vi "FC_Get_Target_Info.vi"(7 "Target":T1, 8 "Error In":errorcluster, 9 "Desired Target":string, 10 "Array of Targets":string[](array[string]), 11 "Target XML":string) -> (0 "error out":errorcluster, 2 "Target Info":string)   [LabVIEW 2013, in "FC_FIRST Client.lvlib"]
doc: "This VI returns all of the information about a specified target"
uses:
  FC_FIRST Client.lvlib
  FC_Target.ctl
  <vilib>/regexp/Match Regular Expression.xnode
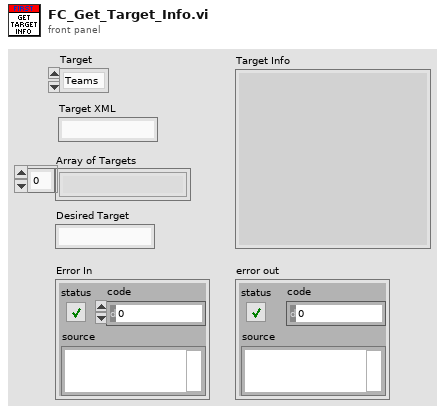
[diagram p1: front panel]
types:
  T1 = typedef "FC_FIRST Client.lvlib/FC_Target.ctl" = enum16{"Teams", "Competitions"}
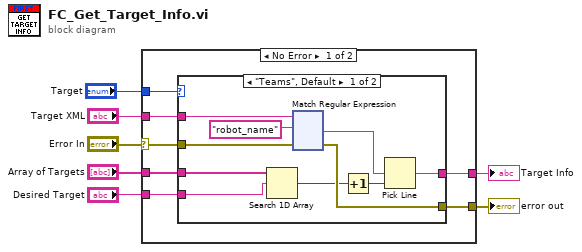
[diagram p0: block diagram]
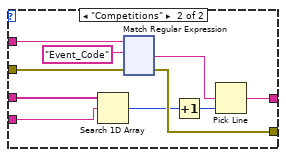
[diagram p2: hidden frame]
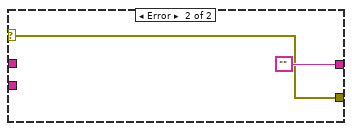
[diagram p3: hidden frame]
diagram:
  n1 = case shown="No Error" "Error In" {
    selector: "Error In" -> [w9 w257]
    tunnel: [w14 w257] -> w7
    tunnel: [w13 "" ("output string")] -> w6
    tunnel: "Desired Target" -> [w12 _]
    tunnel: "Array of Targets" -> [w10 _]
    tunnel: "Target XML" -> [w11 _]
    tunnel: "Target" -> [w8 _]
    frame No Error {
      n2 = case shown="\"Teams\", Default" w8 {
        tunnel: [w24 w145] -> w14
        tunnel: [w22 w143] -> w13
        tunnel: w12 -> [w18 w139]
        tunnel: w11 -> [w17 w138]
        tunnel: w10 -> [w16 w137]
        tunnel: w9 -> [w15 w136]
        frame "Teams", Default {
          n3 = Search 1D Array(1D array=w16, element=w18) -> (index of element=w23:i32)  [unwired: 1 in]
          n4 = xnode "Match Regular Expression"("input string"=w17, "regular expression"="robot_name", "error in"=w15) -> ("after match"=w20:string, "error out"=w24:errorcluster)  [unwired: 3 in, 3 out]
          n5 = Increment(x=w23) -> (x+1=w19:i32)
          n6 = Pick Line(multi-line string=w20, line index=w19) -> (output string=w22:string)  [unwired: 1 in]
        }
        frame "Competitions" {
          n7 = Search 1D Array(1D array=w137, element=w139) -> (index of element=w144:i32)  [unwired: 1 in]
          n8 = xnode "Match Regular Expression"("input string"=w138, "regular expression"="Event_Code", "error in"=w136) -> ("after match"=w141:string, "error out"=w145:errorcluster)  [unwired: 3 in, 3 out]
          n9 = Increment(x=w144) -> (x+1=w140:i32)
          n10 = Pick Line(multi-line string=w141, line index=w140) -> (output string=w143:string)  [unwired: 1 in]
        }
      }
    }
    frame Error {
    }
  }
  "error out" <- w7
  "Target Info" <- w6
